vi "Digit to color convert.vi"(4 "Digit":T1) -> (1 "Color Box":u32(colorbox))   [LabVIEW 2018]
uses:
  Digit.ctl
  Resistor Band Colors/Resistor Band Colors.lvlib
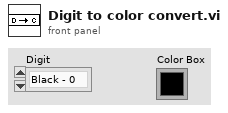
[diagram p1: front panel]
types:
  T1 = typedef "Digit.ctl" = enum16{"Black - 0", "Brown - 1", "Red - 2", "Orange - 3", "Yellow - 4", "Green - 5", "Blue - 6", "Violet - 7", "Grey - 8", "White - 9"}
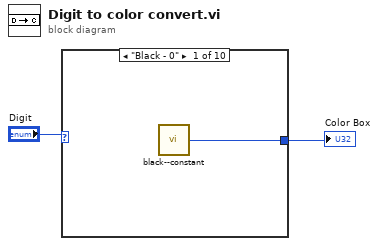
[diagram p0: block diagram]
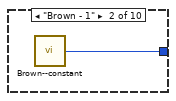
[diagram p2: hidden frame]
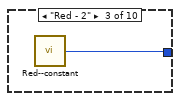
[diagram p3: hidden frame]
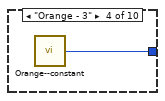
[diagram p4: hidden frame]
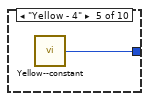
[diagram p5: hidden frame]
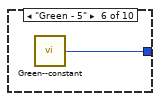
[diagram p6: hidden frame]
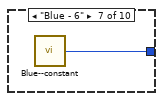
[diagram p7: hidden frame]
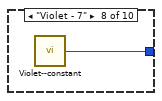
[diagram p8: hidden frame]
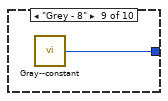
[diagram p9: hidden frame]
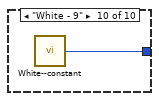
[diagram p10: hidden frame]
diagram:
  n1 = case shown="\"Black - 0\"" "Digit" {
    tunnel: [w3 w4 w5 w6 w7 w8 w9 w10 w11 w12] -> w1
    frame "Black - 0" {
      n2 = call "black--constant.vi"() -> ("Color"=w3:u32)  [unwired: 5 in]
    }
    frame "Brown - 1" {
      n3 = call "Brown--constant.vi"() -> ("Color"=w4:u32)  [unwired: 5 in]
    }
    frame "Red - 2" {
      n4 = call "Red--constant.vi"() -> ("Color"=w5:u32)  [unwired: 5 in]
    }
    frame "Orange - 3" {
      n5 = call "Orange--constant.vi"() -> ("Color"=w6:u32)  [unwired: 5 in]
    }
    frame "Yellow - 4" {
      n6 = call "Yellow--constant.vi"() -> ("Color"=w7:u32)  [unwired: 5 in]
    }
    frame "Green - 5" {
      n7 = call "Green--constant.vi"() -> ("Color"=w8:u32)  [unwired: 5 in]
    }
    frame "Blue - 6" {
      n8 = call "Blue--constant.vi"() -> ("Color"=w9:u32)  [unwired: 5 in]
    }
    frame "Violet - 7" {
      n9 = call "Violet--constant.vi"() -> ("Color"=w10:u32)  [unwired: 5 in]
    }
    frame "Grey - 8" {
      n10 = call "Gray--constant.vi"() -> ("Color"=w11:u32)  [unwired: 5 in]
    }
    frame "White - 9" {
      n11 = call "White--constant.vi"() -> ("Color"=w12:u32)  [unwired: 5 in]
    }
  }
  "Color Box" <- w1
